vi "Direction_detection.vi"() -> ()   [LabVIEW 2016]
uses:
  <vilib>/rvi/interface/nirviOpenFPGA/nirviOpenFPGA.xnode
  FPGA Bitfiles/IntelliRupter2_FPGATarget.lvbitx
  <vilib>/rvi/interface/nirviReadWriteControl/nirviReadWriteControl.xnode
  <vilib>/addons/Electrical Power/Basic/NI_EP_Basic.lvlib
  <vilib>/addons/Electrical Power/Basic/Measurement/RMS (N Channels).vi
  <vilib>/rvi/interface/nirviCloseFPGA/nirviCloseFPGA.xnode
  <vilib>/addons/Electrical Power/Basic/Measurement/Power (1 Channel).vi
  <vilib>/FPGAPlugInAG/cRIO-9039 (Sync)/niLvFpga_Open_cRIO-9039 (Sync).vi
  <vilib>/rvi/interface/common/dynamic/niFpgaDynamicAddResources.vi
  <vilib>/rvi/interface/Simulation/niFpgaSimulationCallBeginRW.vi
  <vilib>/rvi/errors/niLvFpgaAdjustHostInterfaceError.vi
  <vilib>/FPGAPlugInAG/Dynamic/niLvFpga_Close_Dynamic.vi
  <vilib>/addons/Electrical Power/Basic/Measurement/subVIs/basic_Power Value.ctl
panel:
  out "Power":dbl(graph)
  out "Voltage":waveform(sgl)(graph)
  out "Current":waveform(sgl)(graph)
  out "power value":T1
  in  "Relay7":bool
  in  "stop":bool
  out "half cycle (samples)":i32=96
  out "basic calc interval":u16=38
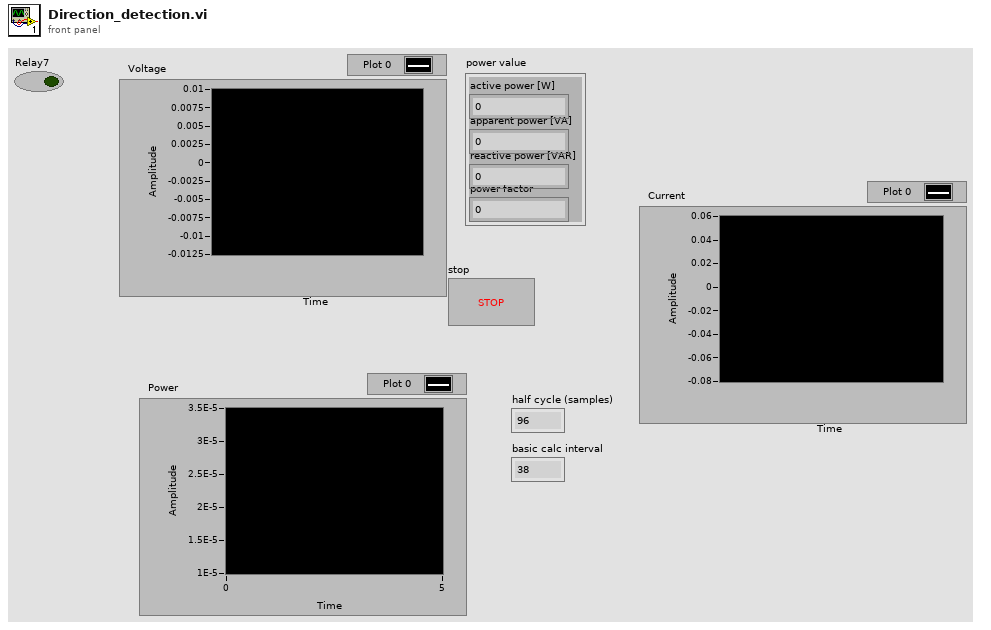
[diagram p1: front panel]
types:
  T1 = typedef "NI_EP_Basic.lvlib/basic_Power Value.ctl" = cluster{"active power [W]":dbl, "apparent power [VA]":dbl, "reactive power [VAR]":dbl, "power factor":dbl}
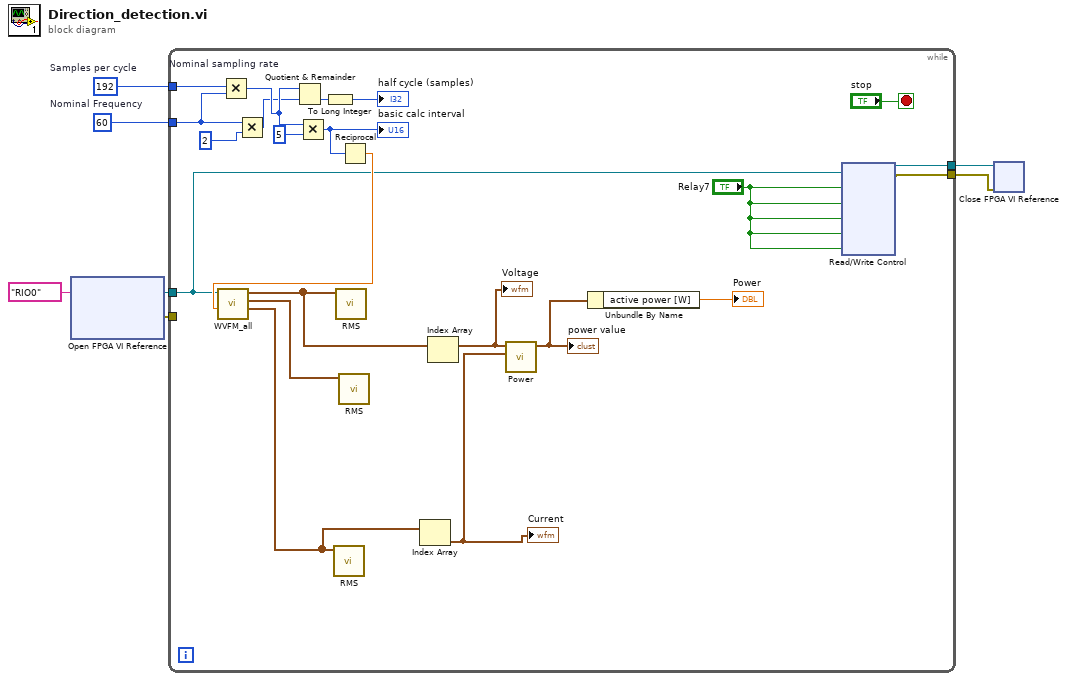
[diagram p0: block diagram]
diagram:
  w3 = 192  # Samples per cycle
  w4 = 60  # Nominal Frequency
  n1 = xnode "Open FPGA VI Reference"("resource name"=tag "RIO0") -> ("FPGA VI Reference Out"=w7:refnum<k20>, "error out"=w6:errorcluster)  [unwired: 1 in]
  n2 = while {
    tunnel: w7 -> [w18]
    tunnel: w6 -> [_]
    tunnel: w4 -> [w22]
    tunnel: w3 -> [w21]
    tunnel: [w16] -> w2
    tunnel: [w15] -> w1
    stop <- "stop" stop-if-true
    n3 = Multiply "Nominal sampling rate"(x=w21, y=w22) -> (x*y=w28:i32)
    n4 = Multiply(x=w22, y=2) -> (x*y=w24:i32)
    n5 = Quotient & Remainder(x=w28, y=w24) -> (floor(x/y)=w26:i32)  [unwired: 1 out]
    n6 = Multiply(x=w28, y=u16 5) -> (x*y=w29:i32)
    "basic calc interval" <- w29
    n7 = To Long Integer(number=w26) -> (32bit integer=→"half cycle (samples)":i32)
    n8 = Reciprocal(x=w29) -> (1/x=w19:dbl)
    n9 = call "WVFM_all.vi"("dt"=w19, "FPGA VI Reference"=w18) -> ("I array"=w13:waveform(sgl)[], "VR array"=w17:waveform(sgl)[], "VL array"=w14:waveform(sgl)[])  [unwired: 6 in]
    n10 = call-poly <vilib>:"RMS.vi"("waveforms"=w13) -> ()  [unwired: 9 in, 2 out]
    n11 = call-poly <vilib>:"RMS.vi"("waveforms"=w14) -> ()  [unwired: 9 in, 2 out]
    n12 = call-poly <vilib>:"RMS.vi"("waveforms"=w17) -> ()  [unwired: 9 in, 2 out]
    n13 = Index Array(array=w13) -> (element=w11:waveform(sgl))  [unwired: 1 in]
    "Current" <- w11
    n14 = Index Array(array=w14) -> (element=w10:waveform(sgl))  [unwired: 1 in]
    "Voltage" <- w10
    n15 = call-poly <vilib>:"Power.vi"("current waveform"=w11, "voltage waveform"=w10) -> ("power value"=w9:T1)  [unwired: 8 in, 1 out]
    "power value" <- w9
    n16 = Unbundle By Name(w9) -> ("active power [W]"=→"Power":dbl)
    n17 = xnode "Read/Write Control"("FPGA VI Reference In"=w18, "Relay8"="Relay7", "Relay1"="Relay7", "Relay2"="Relay7", "Relay3"="Relay7", "Relay5"="Relay7") -> ("FPGA VI Reference Out"=w16:refnum<k20>, "error out"=w15:errorcluster)  [unwired: 1 in]
  }
  n18 = xnode "Close FPGA VI Reference"("FPGA VI Reference In"=w2, "error in"=w1) -> ()  [unwired: 1 out]
